vi "Q Driver_Review.vi"(6 "Q Options":T2, 8 "error in (no error)":errorcluster, 10 "EN Q N":T1[](array[typedef]), 11 "En Q":T1) -> (0 "error out":errorcluster, 3 "De Q":T1)   [LabVIEW 2017]
uses:
  Controls/Review_Q options.ctl
  Controls/Review EnQ.ctl
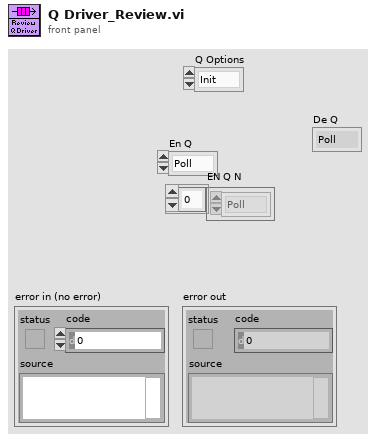
[diagram p1: front panel]
types:
  T1 = typedef "Review EnQ.ctl" = enum16{"Poll", "Init", "Connect", "Close", "Generate Query", "Update", "Take All Reference", "Check Tables & Create", "Read DB", "Export to Pdf", "Export to Csv", "Error", "Exit"}
  T2 = typedef "Review_Q options.ctl" = enum16{"Init", "En Q", "EN Q N", "EN Q Stack", "EN Q Stack N", "De Q", "Flush", "Close"}
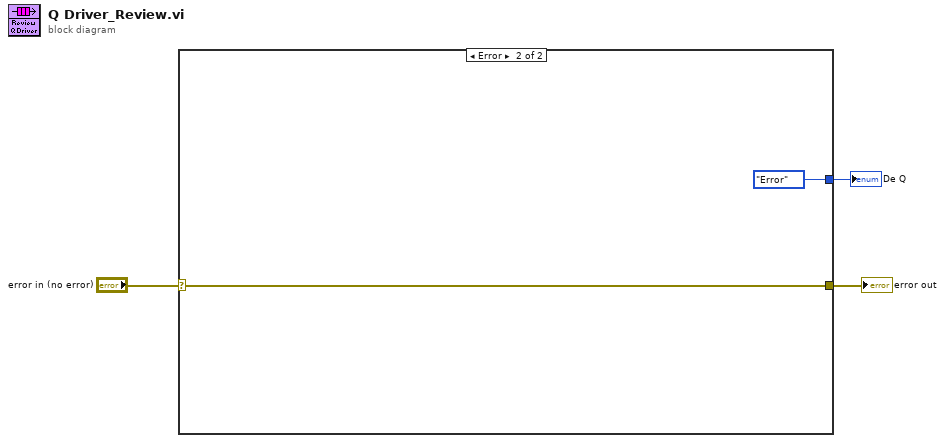
[diagram p0: block diagram]
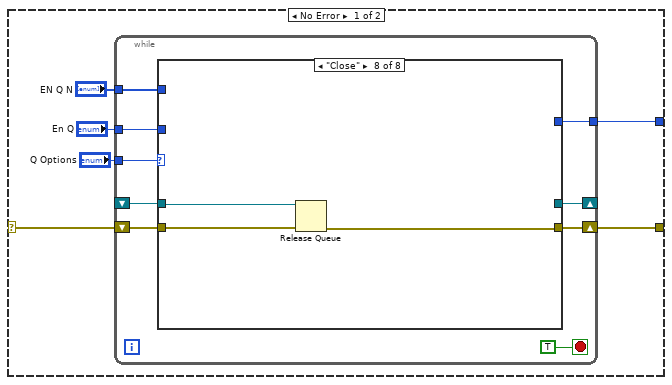
[diagram p2: hidden frame]
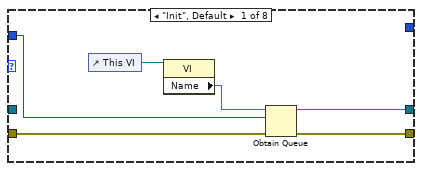
[diagram p3: hidden frame]
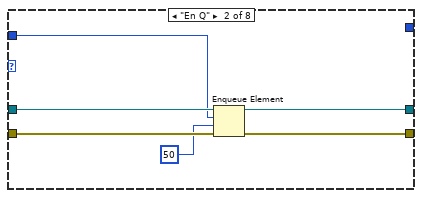
[diagram p4: hidden frame]
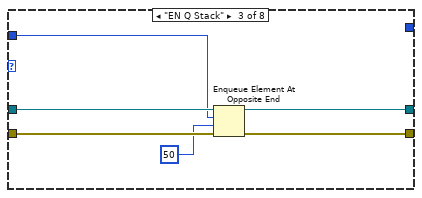
[diagram p5: hidden frame]
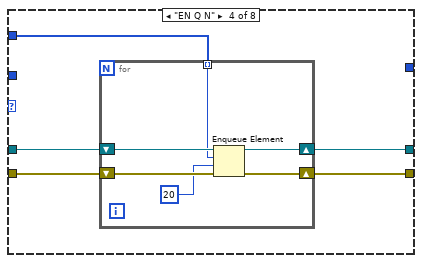
[diagram p6: hidden frame]
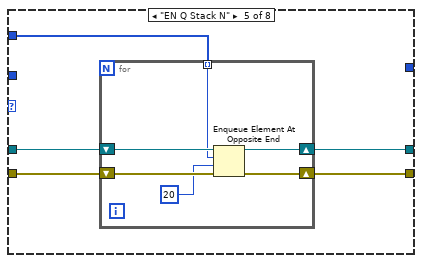
[diagram p7: hidden frame]
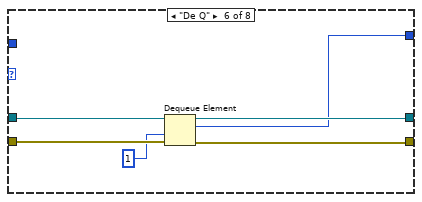
[diagram p8: hidden frame]
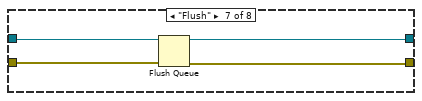
[diagram p9: hidden frame]
diagram:
  n1 = case shown="Error" "error in (no error)" {
    selector: "error in (no error)" -> [w9 w73]
    tunnel: [w8 w73] -> w2
    tunnel: [w4 Review_EnQ."Error" ("En Q")] -> w1
    frame No Error {
      n2 = while {
        shift-right: [w13] -> w8
        shift-left: w9 -> [w17]
        tunnel: "Q Options" -> [w16]
        tunnel: "En Q" -> [w15]
        tunnel: "EN Q N" -> [w14]
        shift-right: [w12] -> _
        shift-left: _ -> [w11]
        tunnel: [w10] -> w4
        stop <- TRUE stop-if-true
        n3 = case shown="\"Close\"" w16 {
          tunnel: w17 -> [w24 w29 w35 w40 w51 w63 w67 w70]
          tunnel: w15 -> [w21 w25 w31 _ _ _ _ _]
          tunnel: w14 -> [_ _ _ w37 w48 _ _ _]
          tunnel: [w23 w28 w34 w39 w50 w62 w66 w69] -> w13
          tunnel: [w22 w27 w33 w38 w49 w61 w65 _] -> w12
          tunnel: w11 -> [_ w30 w36 w41 w52 w64 w68 w71]
          tunnel: [_ _ _ _ _ w59 _ _] -> w10
          frame "Init", Default {
            n4 = control-ref of="This VI"() -> (w20:refnum<vi>)
            n5 = property class="VI"(reference=w20) -> ("Name"=w19:string)  [unwired: 1 in, 2 out]
            n6 = Obtain Queue(name (unnamed)=w19, element data type=w21, error in (no error)=w24) -> (queue out=w22:refnum<queue>, error out=w23:errorcluster)  [unwired: 2 in, 1 out]
          }
          frame "En Q" {
            n7 = Enqueue Element(queue=w30, element=w25, timeout in ms (-1)=50, error in (no error)=w29) -> (queue out=w27:refnum<queue>, error out=w28:errorcluster)  [unwired: 1 out]
          }
          frame "EN Q Stack" {
            n8 = Enqueue Element At Opposite End(queue=w36, element=w31, timeout in ms (-1)=50, error in (no error)=w35) -> (queue out=w33:refnum<queue>, error out=w34:errorcluster)  [unwired: 1 out]
          }
          frame "EN Q N" {
            n9 = for {
              shift-right: [w44] -> w38
              shift-left: w41 -> [w47]
              shift-right: [w45] -> w39
              shift-left: w40 -> [w46]
              tunnel: w37 -> [w42] mode=indexing
              n10 = Enqueue Element(queue=w47, element=w42, timeout in ms (-1)=20, error in (no error)=w46) -> (queue out=w44:refnum<queue>, error out=w45:errorcluster)  [unwired: 1 out]
            }
          }
          frame "EN Q Stack N" {
            n11 = for {
              shift-right: [w55] -> w49
              shift-left: w52 -> [w58]
              shift-right: [w56] -> w50
              shift-left: w51 -> [w57]
              tunnel: w48 -> [w53] mode=indexing
              n12 = Enqueue Element At Opposite End(queue=w58, element=w53, timeout in ms (-1)=20, error in (no error)=w57) -> (queue out=w55:refnum<queue>, error out=w56:errorcluster)  [unwired: 1 out]
            }
          }
          frame "De Q" {
            n13 = Dequeue Element(queue=w64, timeout in ms (-1)=1, error in (no error)=w63) -> (queue out=w61:refnum<queue>, element=w59:T1, error out=w62:errorcluster)  [unwired: 1 out]
          }
          frame "Flush" {
            n14 = Flush Queue(queue=w68, error in (no error)=w67) -> (queue out=w65:refnum<queue>, error out=w66:errorcluster)  [unwired: 1 out]
          }
          frame "Close" {
            n15 = Release Queue(queue=w71, error in (no error)=w70) -> (error out=w69:errorcluster)  [unwired: 1 in, 2 out]
          }
        }
      }
    }
    frame Error {
    }
  }
  "error out" <- w2
  "De Q" <- w1
